vi "toggle_enable.vi"(8 "error in (no error)":errorcluster, 11 "reference":refnum<vi>) -> (0 "error out":errorcluster)   [LabVIEW 2017]
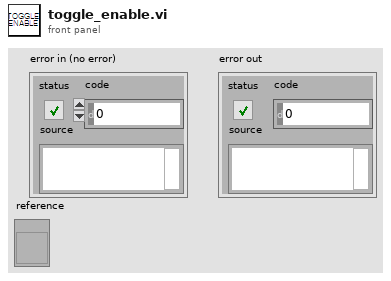
[diagram p1: front panel]
types:
  T1 = enum8{"Enabled", "Disabled", "Disabled and Grayed Out"}
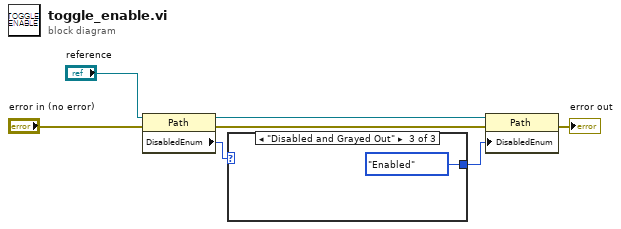
[diagram p0: block diagram]
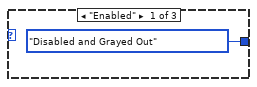
[diagram p2: hidden frame]
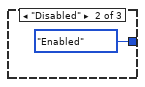
[diagram p3: hidden frame]
diagram:
  n1 = property on="Property Node" class="Path"(reference="reference", error in="error in (no error)") -> (reference out=w4:refnum<vi>, error out=w1:errorcluster, "DisabledEnum"=w3:T1)
  n2 = case shown="\"Disabled and Grayed Out\"" w3 {
    tunnel: [T1."Disabled and Grayed Out" ("Disabled") T1."Enabled" ("Disabled") T1."Enabled" ("Disabled")] -> w6
    frame "Enabled" {
    }
    frame "Disabled" {
    }
    frame "Disabled and Grayed Out" {
    }
  }
  n3 = property on="Property Node" class="Path"(reference=w4, error in=w1, "DisabledEnum"=w6) -> (error out=→"error out":errorcluster)  [unwired: 1 out]
